vi "Devices Not On.vi"(8 "All Devices Core Info":string[][](array[string]), 9 "Experiment":string, 10 "Preset Table Control":string[][](array[string]), 11 "queue":refnum<queue>) -> (1 "Preset Devices Not Alive":string[](array[string]), 3 "Devices Not alive":string[](array[string]))   [LabVIEW 2020]
uses:
  Preset Query Enum.ctl
  9841071b-ee7c-4f89-9e1d-a924ed6892d8.vi
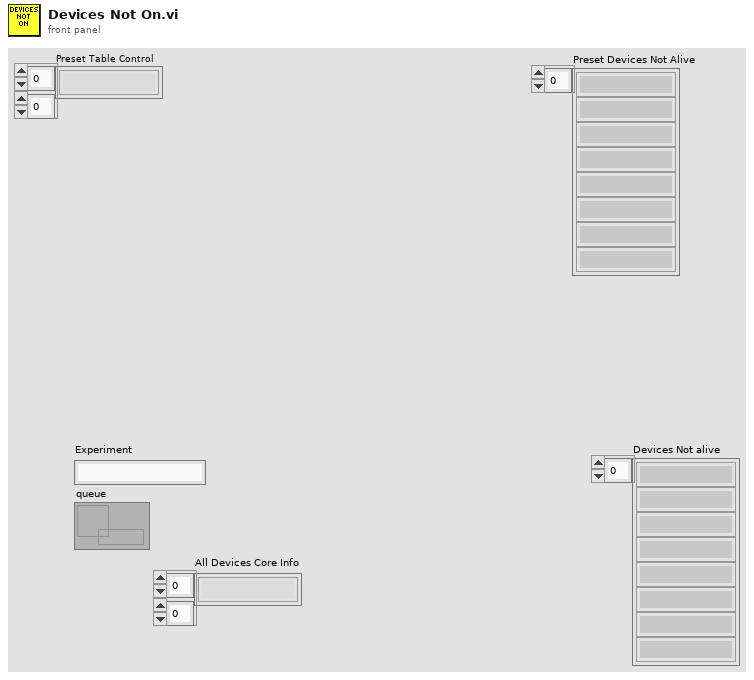
[diagram p1: front panel]
types:
  T1 = typedef "Preset Query Enum.ctl" = enum16{"Get Locations", "Get all IPs and MACs", "Get classes", "Get expt variables to set at scanstart for particular device", "Get expt devices and variables with start values", "Get expt devices and variables (with data to get)", "Get expt devices with data to get", "Get Expt devices and GUIs", "Get all devices basic properties", "Get Virtual Devices Core Info", "Get Expt names", "Get experiment basic properties", "Get experiment alarm variables", "Get MC Ports", "Get device network comm port", "Get devicetype lvclass path", "Get basic device properties", "Get Init Order", "Get all setable variables of a device", "Get device variable aliases", "Get force values of all settable variables", "Get all variables of a devicetype", "Get all variables of a device", "Get plotter details", "Get Saved Scans", "Get Scan Info", "GetGeneralGUIs", "Get expt for plotter", "Get plotter IDs from expt", "Get all devices", "Get all Virtual Devices", "Get all aliases", "Get variable and device info for Virtual Device", "GetItemLocatorIP", "Get IPs for GUIs", "Get DeviceType from Device", "GetLocalPortRange", "GetDevicePresetVariables", "Get Device Configuration", "GetAllPresetNames", "GetAllConfigurationNames", "GetPresetDeviceNames", "GetDeviceAliases", "GetDevicesOfClass"}
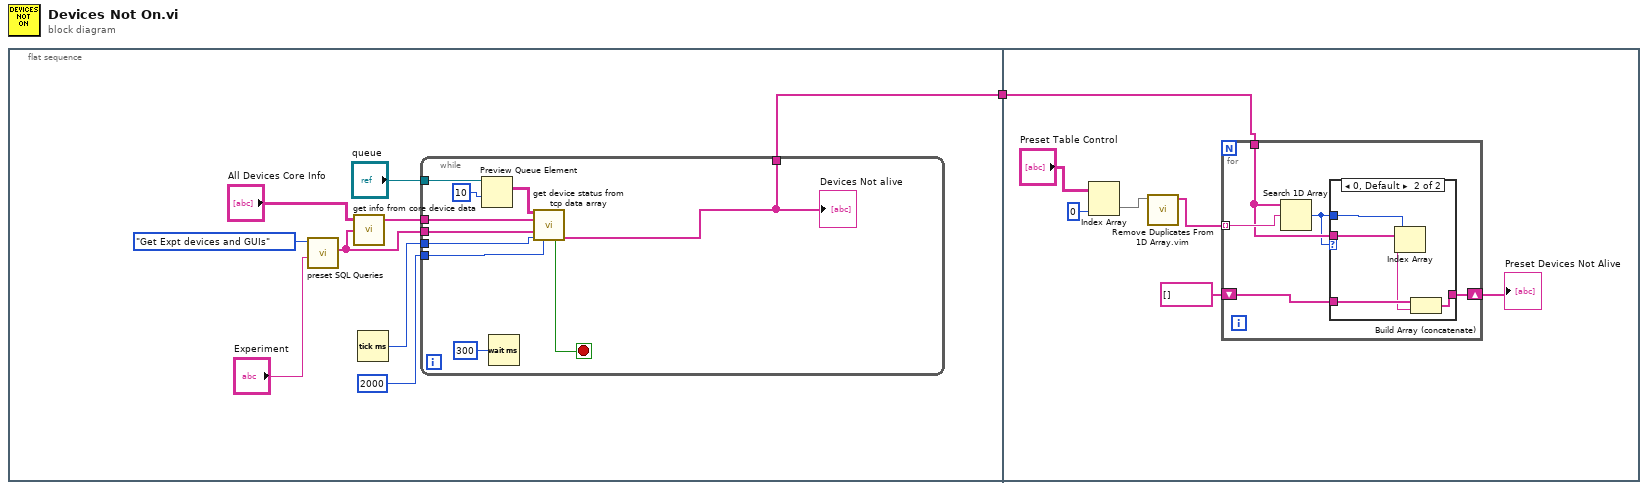
[diagram p0: block diagram]
diagram:
  n1 = flat-sequence {
    tunnel: [w2] -> w1
    tunnel: w1 -> [w23]
    frame #0 {
      n2 = call "preset SQL Queries.vi"("Expt name / MCIP/ Variable/Preset Name"="Experiment", "Preset Query"=Preset_Query_Enum."Get Expt devices and GUIs") -> ("1st column 1st data"=w3:string[])  [unwired: 7 in, 2 out]
      n3 = call "get info from core device data.vi"("devices to get data from"=w3, "All Devices Core Info"="All Devices Core Info") -> ("IP Addresses"=w7:string[])  [unwired: 2 in, 1 out]
      n4 = Tick Count (ms)() -> (millisecond timer value=w5:u32)
      n5 = while {
        tunnel: w7 -> [w19]
        tunnel: w3 -> [w18]
        tunnel: "queue" -> [w17]
        tunnel: w5 -> [w16]
        tunnel: 2000 ("timeout") -> [w15]
        tunnel: [w11] -> w2
        stop <- w13 stop-if-true
        n6 = Preview Queue Element(queue=w17, timeout in ms (-1)=10) -> (element=w20:string[][])  [unwired: 1 in, 3 out]
        n7 = Wait (ms)(milliseconds to wait=u32 300) -> ()  [unwired: 1 out]
        n8 = call "get device status from tcp data array.vi"("TCP Device status data"=w20, "IP Addresses in"=w19, "Filtered Device List"=w18, "input ms timer value"=w16, "timeout"=w15) -> ("exit loop"=w13:bool, "Devices Not alive"=w11:string[])  [unwired: 3 in, 6 out]
        "Devices Not alive" <- w11
      }
    }
    frame #1 {
      n9 = Index Array(array="Preset Table Control", index (col)=0 ("disabled index (col)")) -> (element=w25:string[])  [unwired: 1 in]
      n10 = call "Remove Duplicates From 1D Array.vim"("array"=w25) -> ("array with duplicates removed"=w24:string[])  [unwired: 10 in]
      n11 = for {
        tunnel: w24 -> [w32] mode=indexing
        tunnel: w23 -> [w31]
        shift-right: [w30] -> w21
        shift-left: string[] [] -> [w29]
        n12 = Search 1D Array(1D array=w31, element=w32) -> (index of element=w28:i32)  [unwired: 1 in]
        n13 = case shown="0, Default" w28 {
          tunnel: w31 -> [_ w38]
          tunnel: [w33 w37] -> w30
          tunnel: w29 -> [w33 w36]
          tunnel: w28 -> [_ w35]
          frame -1 {
          }
          frame 0, Default {
            n14 = Index Array(array=w38, index=w35) -> (element=w34:string)
            n15 = Build Array (concatenate)(w36, w34) -> (w37:string[])
          }
        }
      }
      "Preset Devices Not Alive" <- w21
    }
  }
